vi "CreateBoard.vi"(11 "Squares type":T1[][](array[typedef])) -> (3 "Board":u16[][](array[numeric]))   [LabVIEW 2019]
doc: "This VI creates board image from information about squares type"
uses:
  #typedef_SquareType.ctl
  #typedef_Color.ctl
  #typedef_Piece.ctl
  #typedef_PieceType.ctl
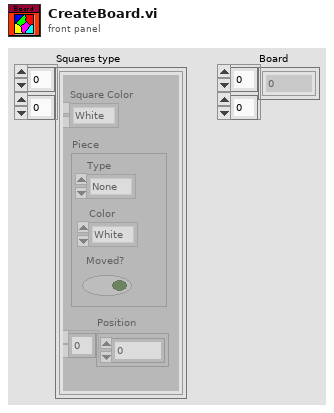
[diagram p1: front panel]
types:
  T1 = typedef "#typedef_SquareType.ctl" = cluster{"Square Color":T2, "Position":i32[], "Piece":T3}
  T2 = typedef "#typedef_Color.ctl" = enum16{"White", "Black"}
  T3 = typedef "#typedef_Piece.ctl" = cluster{"Type":T4, "Color":T2, "Moved?":bool}
  T4 = typedef "#typedef_PieceType.ctl" = enum16{"None", "Pawn", "Knight", "Bishop", "Rook", "Queen", "King"}
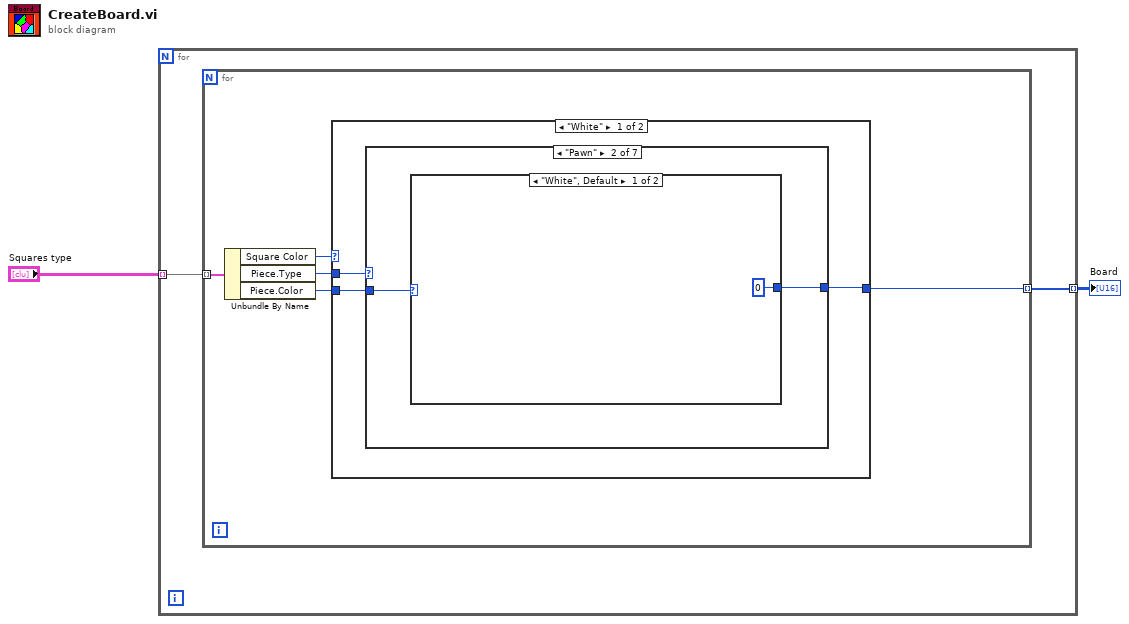
[diagram p0: block diagram]
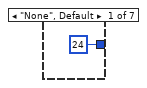
[diagram p2: hidden frame]
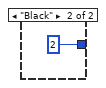
[diagram p3: hidden frame]
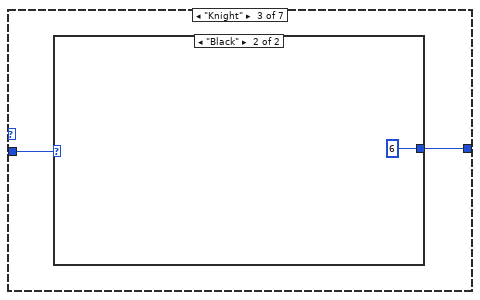
[diagram p4: hidden frame]
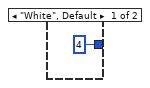
[diagram p5: hidden frame]
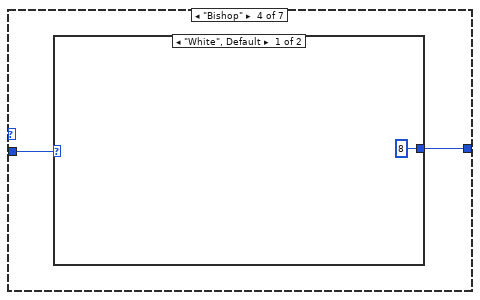
[diagram p6: hidden frame]
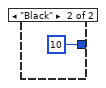
[diagram p7: hidden frame]
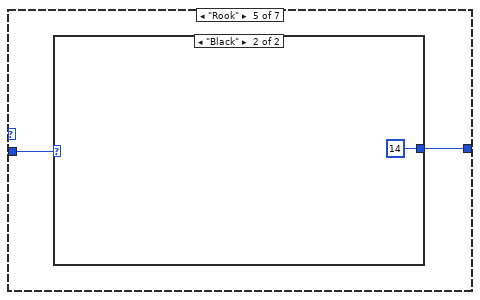
[diagram p8: hidden frame]
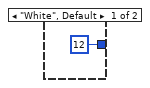
[diagram p9: hidden frame]
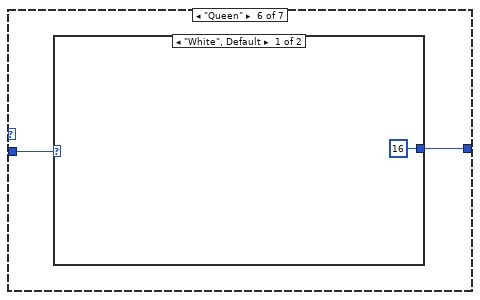
[diagram p10: hidden frame]
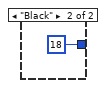
[diagram p11: hidden frame]
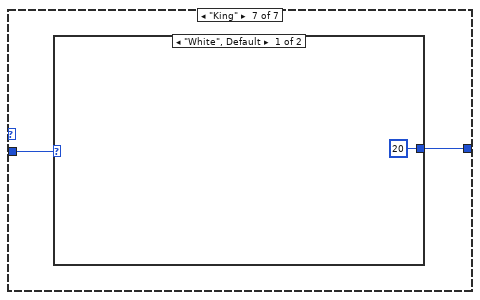
[diagram p12: hidden frame]
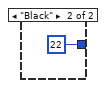
[diagram p13: hidden frame]
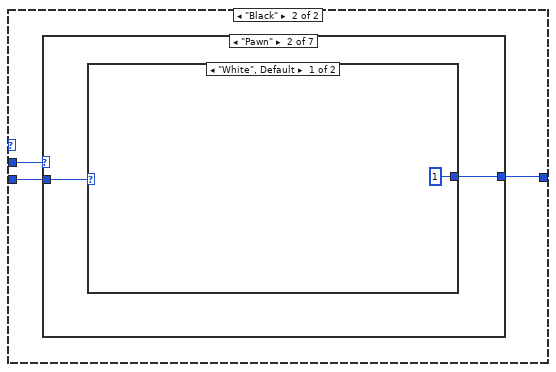
[diagram p14: hidden frame]
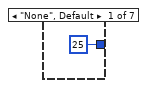
[diagram p15: hidden frame]
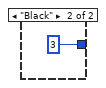
[diagram p16: hidden frame]
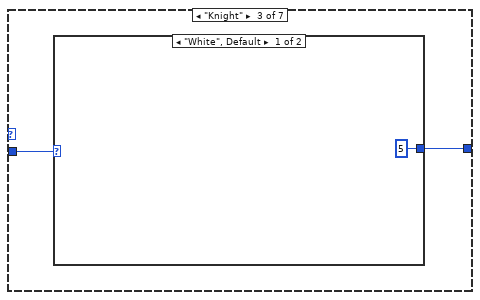
[diagram p17: hidden frame]
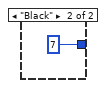
[diagram p18: hidden frame]
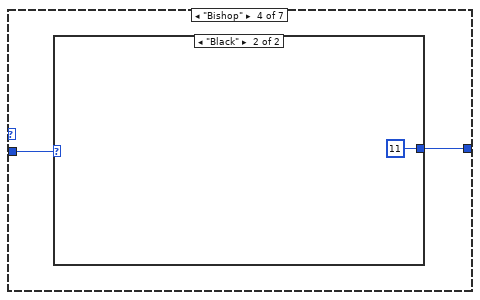
[diagram p19: hidden frame]
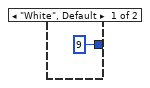
[diagram p20: hidden frame]
diagram:
  n1 = for {
    tunnel: "Squares type" -> [w4] mode=indexing
    tunnel: [w3] -> w2 mode=indexing
    n2 = for {
      tunnel: w4 -> [w9] mode=indexing
      tunnel: [w5] -> w3 mode=indexing
      n3 = Unbundle By Name(w9) -> ("Square Color"=w8:T2, "Piece.Type"=w7:T4, "Piece.Color"=w6:T2)
      n4 = case shown="\"White\"" w8 {
        tunnel: w7 -> [w12 w40]
        tunnel: w6 -> [w11 w39]
        tunnel: [w10 w38] -> w5
        frame "White" {
          n5 = case shown="\"Pawn\"" w12 {
            tunnel: w11 -> [_ w15 w19 w23 w27 w31 w35]
            tunnel: [u16 24 ("Square Look") w14 w18 w22 w26 w30 w34] -> w10
            frame "None", Default {
            }
            frame "Pawn" {
              n6 = case shown="\"White\", Default" w15 {
                tunnel: [u16 0 ("Square Look") u16 2 ("Square Look")] -> w14
                frame "White", Default {
                }
                frame "Black" {
                }
              }
            }
            frame "Knight" {
              n7 = case shown="\"Black\"" w19 {
                tunnel: [u16 4 ("Square Look") u16 6 ("Square Look")] -> w18
                frame "White", Default {
                }
                frame "Black" {
                }
              }
            }
            frame "Bishop" {
              n8 = case shown="\"White\", Default" w23 {
                tunnel: [u16 8 ("Square Look") u16 10 ("Square Look")] -> w22
                frame "White", Default {
                }
                frame "Black" {
                }
              }
            }
            frame "Rook" {
              n9 = case shown="\"Black\"" w27 {
                tunnel: [u16 12 ("Square Look") u16 14 ("Square Look")] -> w26
                frame "White", Default {
                }
                frame "Black" {
                }
              }
            }
            frame "Queen" {
              n10 = case shown="\"White\", Default" w31 {
                tunnel: [u16 16 ("Square Look") u16 18 ("Square Look")] -> w30
                frame "White", Default {
                }
                frame "Black" {
                }
              }
            }
            frame "King" {
              n11 = case shown="\"White\", Default" w35 {
                tunnel: [u16 20 ("Square Look") u16 22 ("Square Look")] -> w34
                frame "White", Default {
                }
                frame "Black" {
                }
              }
            }
          }
        }
        frame "Black" {
          n12 = case shown="\"Pawn\"" w40 {
            tunnel: w39 -> [_ w43 w47 w51 w55 w59 w63]
            tunnel: [u16 25 ("Square Look") w42 w46 w50 w54 w58 w62] -> w38
            frame "None", Default {
            }
            frame "Pawn" {
              n13 = case shown="\"White\", Default" w43 {
                tunnel: [u16 1 ("Square Look") u16 3 ("Square Look")] -> w42
                frame "White", Default {
                }
                frame "Black" {
                }
              }
            }
            frame "Knight" {
              n14 = case shown="\"White\", Default" w47 {
                tunnel: [u16 5 ("Square Look") u16 7 ("Square Look")] -> w46
                frame "White", Default {
                }
                frame "Black" {
                }
              }
            }
            frame "Bishop" {
              n15 = case shown="\"Black\"" w51 {
                tunnel: [u16 9 ("Square Look") u16 11 ("Square Look")] -> w50
                frame "White", Default {
                }
                frame "Black" {
                }
              }
            }
            frame "Rook" {
              n16 = case shown="\"White\", Default" w55 {
                tunnel: [u16 13 ("Square Look") u16 15 ("Square Look")] -> w54
                frame "White", Default {
                }
                frame "Black" {
                }
              }
            }
            frame "Queen" {
              n17 = case shown="\"Black\"" w59 {
                tunnel: [u16 17 ("Square Look") u16 19 ("Square Look")] -> w58
                frame "White", Default {
                }
                frame "Black" {
                }
              }
            }
            frame "King" {
              n18 = case shown="\"White\", Default" w63 {
                tunnel: [u16 21 ("Square Look") u16 23 ("Square Look")] -> w62
                frame "White", Default {
                }
                frame "Black" {
                }
              }
            }
          }
        }
      }
    }
  }
  "Board" <- w2
